vi "Compute Motor Instantaneous Values.vi"(9 "Initial motor rpm":dbl, 11 "Motor Type":T3=enum."775 pro") -> ()   [LabVIEW 2020]
uses:
  Motor Type.ctl
  <vilib>/addons/Control Design/_Model Construction/Model Typedefs.llb/CD State Space Model (MIMO).ctl
  <vilib>/addons/Control Design/_Model Construction/Model Typedefs.llb/CD General Elements.ctl
  <vilib>/addons/Control Design/_Model Construction/Model Creation.llb/Model Creation SubVI/cd_Create Symbolic State Space Model.vi
  <vilib>/addons/Control Design/_Model Construction/NI_LinSys_Model Creation.lvlib
  <vilib>/addons/Control Design/_Model Construction/NI_LinSys_Model Typedefs.lvlib
panel:
  out "State Space Model":T1 {"Transport Delay" format="%.2f"; "D" format="%#.2g"; "C" format="%#.2g"; "B" format="%#.2g"; "A" format="%#.2g"; "properties"."Sampling Time" format="%#.6p"; "properties"."Output Delays" format="%.4f"; "properties"."Input Delays" format="%.4f"}
  in  "Variables":cluster{"Name":string, " Value":dbl}[](array[cluster])=[{"Name"="J", " Value"=10.0}, {"Name"="G", " Value"=0.0}, {"Name"="kv", " Value"=20.0}, {"Name"="R", " Value"=50.0}, {"Name"="kt", " Value"=0.0}] {"Value" format="%.2f"}
  in  "Symbolic D":string[][](array[string])=[["0"]]
  in  "Symbolic C":string[][](array[string])=[["1"]]
  in  "Symbolic B":string[][](array[string])=[["G*kt/(R*J)"]]
  in  "Symbolic A":string[][](array[string])=[["-G^2*kt/(kv*R*J)"]]
  out "Chart 2":dbl(graph)
  in  "stop":bool
  in  "timestep":dbl[unit]=0.001 format="%#_3p"
  out "Chart":cluster{"Free Speed":dbl, "Current":dbl[unit]}(graph)
  in  "Effective Voltage":dbl[unit](slide)=4.333333333333336 scale=-13.0..13.0
  # "Recommended use:\nChange the Motor Type, then click the run button in toolbar."
  # "One motor guessing at weight and size\nand without battery droop."
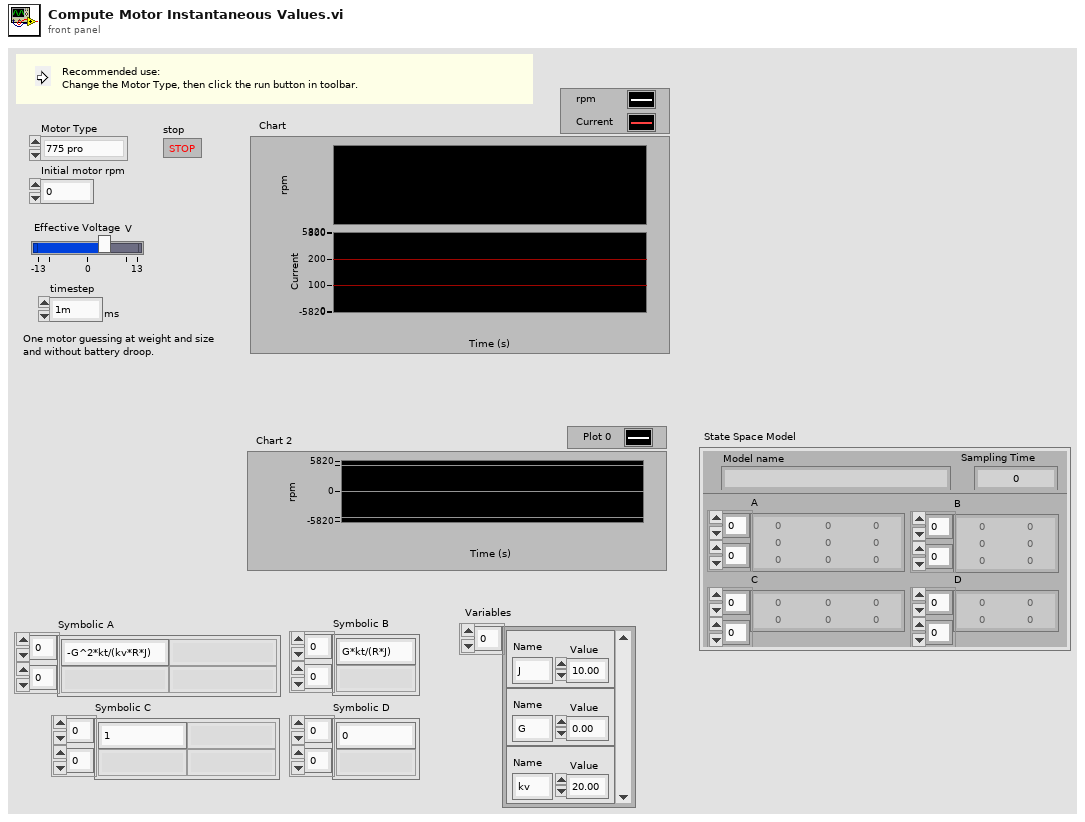
[diagram p1: front panel]
types:
  T1 = typedef "NI_LinSys_Model Typedefs.lvlib/CD State Space Model (MIMO).ctl" = cluster{"properties":T2, "A":dbl[][], "B":dbl[][], "C":dbl[][], "D":dbl[][], "StateNames":string[], "Transport Delay":dbl[][]}
  T2 = typedef "NI_LinSys_Model Typedefs.lvlib/CD General Elements.ctl" = cluster{"Model name":string, "Input names":string[], "Output names":string[], "Input Delays":dbl[], "Output Delays":dbl[], "Sampling Time":dbl, "Notes":string}
  T3 = typedef "Motor Type.ctl" = enum16{"Custom", "775 pro", "CIM", "miniCIM", "Neo", "Neo 550", "Falcon 500"}
  T4 = typedef "Motor Physical Values.ctl" = cluster{"Ratio (out/in)":dbl, "Moment of Inertia (kg m^2)":dbl[unit]}
  T5 = typedef "Motor Operating Values.ctl" = cluster{"Kv":dbl[unit], "R":dbl[unit], "Kt":dbl[unit], "Breaker Size":dbl[unit]}
  T6 = cluster{"Initial motor rpm":dbl, "Current":dbl[unit]}
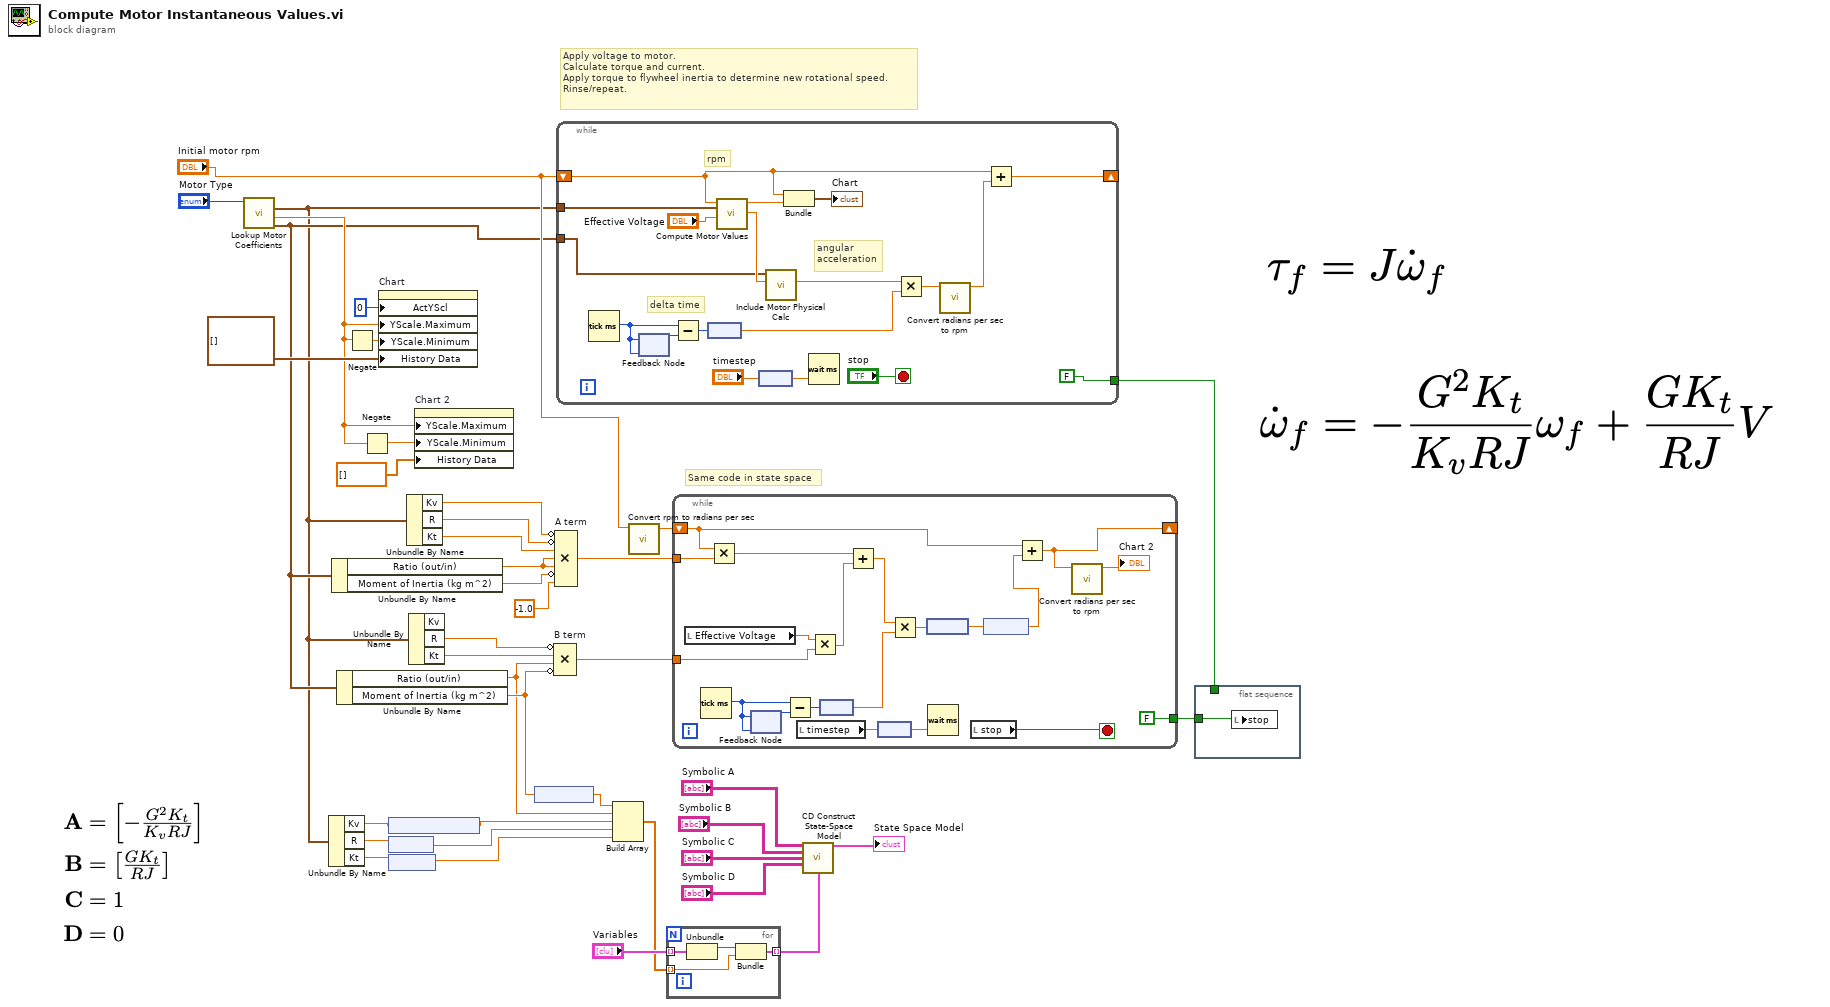
[diagram p0: block diagram]
diagram:
  # "Same code in state space"
  # "Apply voltage to motor.\nCalculate torque and current.\nApply torque to flywheel inertia to determine new rotational speed.\nRinse/repeat."
  n1 = call "Lookup Motor Coefficients.vi"("Motor Type"="Motor Type") -> ("Physical Values"=w14:T4, "Free Speed"=w21:dbl, "Motor Model Values"=w10:T5)  [unwired: 7 in, 1 out]
  n2 = Unbundle By Name(w10) -> ("Kv"=w9:dbl[unit], "R"=w7:dbl[unit], "Kt"=w8:dbl[unit])
  n3 = Unbundle By Name(w14) -> ("Ratio (out/in)"=w36:dbl, "Moment of Inertia (kg m^2)"=w34:dbl[unit])
  n4 = Unbundle By Name(w14) -> ("Ratio (out/in)"=w12:dbl, "Moment of Inertia (kg m^2)"=w13:dbl[unit])
  n5 = Negate(x=w21) -> (-x=w37:dbl)
  n6 = Negate(x=w21) -> (-x=w20:dbl)
  n7 = property on="Chart" class="WFChart (strict)"("ActYScl"=0 ("Active Y Scale"), "YScale.Maximum"=w21, "YScale.Minimum"=w37, "History Data"=cluster{"Free Speed":dbl, "Current":dbl[unit]}[] []) -> ()  [unwired: 2 in, 2 out]
  n8 = node(w9) -> (w6:dbl)
  n9 = node(w7) -> (w5:dbl)
  n10 = node(w8) -> (w4:dbl)
  n11 = Unbundle By Name(w10) -> ("Kv"=w33:dbl[unit], "R"=w32:dbl[unit], "Kt"=w35:dbl[unit])
  n12 = Unbundle By Name(w10) -> ("R"=w29:dbl[unit], "Kt"=w30:dbl[unit])  [unwired: 1 out]
  n13 = property on="Chart 2" class="WFChart (strict)"("YScale.Maximum"=w21, "YScale.Minimum"=w20, "History Data"=dbl[] []) -> ()  [unwired: 2 in, 2 out]
  n14 = node(w13) -> (w11:dbl)
  n15 = Compound Arithmetic op=MULTIPLY "B term"(invert w29, w30, w12, invert w13) -> (w26:dbl[unit])
  n16 = Compound Arithmetic op=MULTIPLY "A term"(invert w33, invert w32, w35, w36, w36, invert w34, -1.0) -> (w28:dbl[unit])
  n17 = while {
    tunnel: w10 -> [w59]
    shift-right: [w57] -> _
    shift-left: "Initial motor rpm" -> [w43]
    tunnel: w14 -> [w42]
    tunnel: [FALSE] -> w23
    stop <- "stop" stop-if-true
    # "angular\nacceleration"
    # "delta time"
    # "rpm"
    n18 = Tick Count (ms)() -> (millisecond timer value=w50:u32)
    n19 = feedback-in #1(w50) -> ()
    n20 = feedback #1(w50) -> (w53:u32)
    n21 = Subtract(x=w50, y=w53) -> (x-y=w52:u32)
    n22 = node(w52) -> (w51:dbl[unit])
    n23 = call "Compute Motor Values.vi"("Effective Motor Voltage"="Effective Voltage", "Motor Model Values"=w59, "motor speed (rpm)"=w43) -> ("Motor Torque"=w45:dbl[unit], "Current"=w49:dbl[unit])  [unwired: 5 in, 2 out]
    n24 = node("timestep") -> (w46:dbl)
    n25 = call "Include Motor Physical Calc.vi"("Motor Torque"=w45, "Physical Values"=w42) -> ("Angular Accel"=w44:dbl[unit])  [unwired: 8 in, 1 out]
    n26 = Bundle("Initial motor rpm"=w43, "Current"=w49) -> (→"Chart":T6)  [unwired: 1 in]
    n27 = Wait (ms)(milliseconds to wait=w46) -> ()  [unwired: 1 out]
    n28 = Multiply(x=w44, y=w51) -> (x*y=w55:dbl[unit])
    n29 = call "Convert radians per sec to rpm.vi"("speed in"=w55) -> ("speed out (rpm)"=w56:dbl)  [unwired: 10 in]
    n30 = Add(x=w43, y=w56) -> (x+y=w57:dbl)
  }
  n31 = Build Array(w11, w12, w6, w5, w4) -> (w3:dbl[])
  n32 = call "Convert rpm to radians per sec.vi"("motor speed (rpm)"="Initial motor rpm") -> ("speed rps"=w25:dbl[unit])  [unwired: 10 in]
  n33 = for {
    tunnel: "Variables" -> [w63] mode=indexing
    tunnel: w3 -> [w61] mode=indexing
    tunnel: [w60] -> w2 mode=indexing
    n34 = Unbundle(w63) -> ("Name"=w62:string)  [unwired: 1 out]
    n35 = Bundle("Name"=w62, "Ratio (out/in)"=w61) -> (w60:cluster{"Name":string, "Ratio (out/in)":dbl})  [unwired: 1 in]
  }
  n36 = while {
    tunnel: w28 -> [w83]
    shift-right: [w69] -> _
    shift-left: w25 -> [w70]
    tunnel: w26 -> [w82]
    tunnel: [FALSE] -> w24
    stop <- w71 stop-if-true
    n37 = local read "Effective Voltage"() -> (w76:dbl[unit])
    n38 = Tick Count (ms)() -> (millisecond timer value=w80:u32)
    n39 = Multiply(x=w70, y=w83) -> (x*y=w81:dbl[unit])
    n40 = feedback #2(w80) -> (w78:u32)
    n41 = feedback-in #2(w80) -> ()
    n42 = Subtract(x=w80, y=w78) -> (x-y=w79:u32)
    n43 = local read "timestep"() -> (w72:dbl[unit])
    n44 = Multiply(x=w76, y=w82) -> (x*y=w75:dbl[unit])
    n45 = node(w79) -> (w77:dbl[unit])
    n46 = Add(x=w81, y=w75) -> (x+y=w74:dbl[unit])
    n47 = node(w72) -> (w73:dbl)
    n48 = Multiply(x=w74, y=w77) -> (x*y=w68:dbl[unit])
    n49 = node(w68) -> (w67:dbl)
    n50 = Wait (ms)(milliseconds to wait=w73) -> ()  [unwired: 1 out]
    n51 = local read "stop"() -> (w71:bool)
    n52 = node(w67) -> (w66:dbl[unit])
    n53 = Add(x=w70, y=w66) -> (x+y=w69:dbl[unit])
    n54 = call "Convert radians per sec to rpm.vi"("speed in"=w69) -> ("speed out (rpm)"=→"Chart 2":dbl)  [unwired: 10 in]
  }
  n55 = call-poly <vilib>:"CD Construct State-Space Model.vi"("Symbolic A"="Symbolic A", "Symbolic B"="Symbolic B", "Symbolic C"="Symbolic C", "Symbolic D"="Symbolic D", "Variables"=w2) -> ("State Space Model"=→"State Space Model":T1)  [unwired: 9 in, 1 out]
  n56 = flat-sequence {
    tunnel: w24 -> [w84]
    tunnel: w23 -> [_]
    frame #0 {
      n57 = local write "stop"(w84) -> ()
    }
  }
